vi "FTW-Connector-Connect.vi"(0 "FTW Actor Connector Type":refnum<class "FTW-Actor-Connector.lvclass">, 5 "Instance Inbox Address":string, 11 "error in":errorcluster) -> (4 "FTW Actor Connector":refnum<class "FTW-Actor-Connector.lvclass">, 15 "error out":errorcluster)   [LabVIEW 2013, in "FTW-Actor-Connector.lvclass"]
doc: "Performs a \"cold call\" to connect to a running Actor Instance at the given Instance Inbox Address. Normally, this method is wrapped by a \"Construct\" method in each specific Actor Connector subclass."
uses:
  FTW-Actor-Connector.lvclass
  socket/FTW-Socket-Type.ctl
  FTW-Actor-Connector.lvclass/FTW-Actor-Connector.ctl
  socket/FTW-Socket.lvclass
panel:
  # "Inputs"
  # "Outputs"
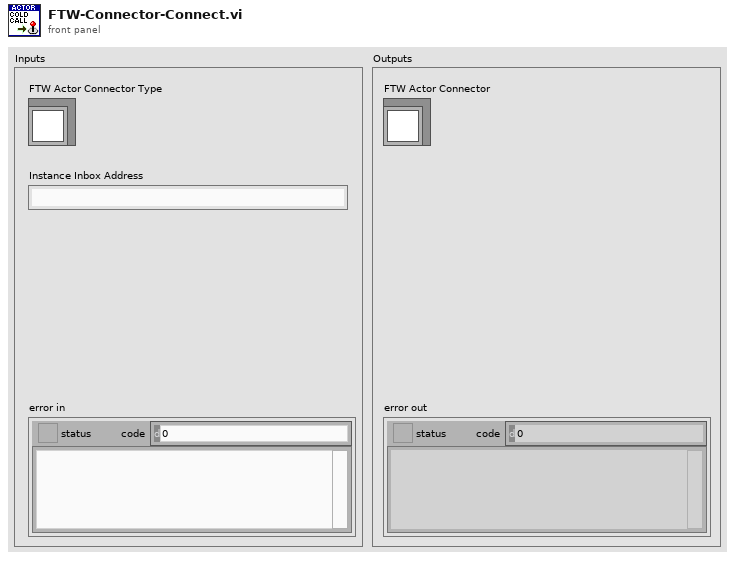
[diagram p1: front panel]
types:
  T1 = typedef "FTW-Socket.lvclass/FTW-Socket-Type.ctl" = enum32{"Server", "Client", "Publisher", "Subscriber", "Pipeline Producer", "Pipeline Consumer", "Surveyor", "Respondent", "Exclusive Pair", "Bus"}
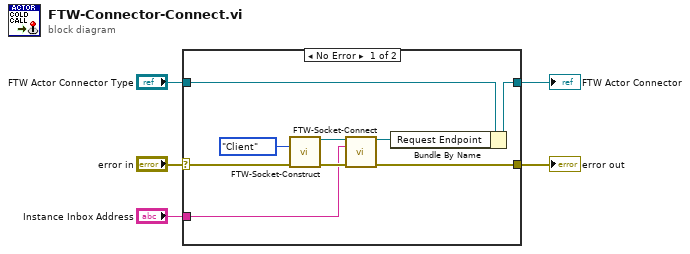
[diagram p0: block diagram]
diagram:
  n1 = case shown="No Error" "error in" {
    selector: "error in" -> [w6 w15]
    tunnel: [w14 w16] -> w5
    tunnel: "FTW Actor Connector Type" -> [w13 w16]
    tunnel: [w9 w15] -> w3
    tunnel: "Instance Inbox Address" -> [w7 _]
    frame No Error {
      n2 = call "FTW-Socket-Construct.vi"("Socket Topology"=FTW-Socket-Type."Client" ("Socket Type"), "error in"=w6) -> ("FTW Socket"=w12:refnum<class "FTW-Socket.lvclass">, "error out"=w10:errorcluster)  [unwired: 12 in]
      n3 = call "FTW-Socket-Connect.vi"("FTW Socket"=w12, "Remote Address"=w7, "error in"=w10) -> ("FTW Socket out"=w8:refnum<class "FTW-Socket.lvclass">, "error out"=w9:errorcluster)  [unwired: 11 in]
      n4 = Bundle By Name(cluster=w13, "Request Endpoint"=w8) -> (w14:refnum<class "FTW-Actor-Connector.lvclass">)
    }
    frame Error {
    }
  }
  "error out" <- w3
  "FTW Actor Connector" <- w5
